vi "Execute.vi"(8 "error in (no error)":errorcluster, 11 "Start Pre-Soak in":refnum<class "Initialize HMI.lvclass">) -> (0 "error out":errorcluster, 3 "Start Pre-Soak out":refnum<class "Initialize HMI.lvclass">)   [LabVIEW 2019, in "Initialize HMI.lvclass"]
uses:
  <vilib>/gpm_packages/@cs/Car-wash/Source/Process Steps/Initialize HMI/Initialize HMI.lvclass
  C:/Program Files/National Instruments/LabVIEW 2019/vi.lib/gpm_packages/@cs/mva-core/Source/IModel/IModel/IModel.lvclass
  C:/Program Files/National Instruments/LabVIEW 2019/vi.lib/ActorFramework/Actor/Actor.lvclass
  <vilib>/gpm_packages/@cs/mva-core/Source/IObserver/IObserver/IObserver.lvclass/IObserver.ctl
  <vilib>/gpm_packages/@cs/mva-core/Source/IModel/IModel/IModel.lvclass/IModel.ctl
  <vilib>/gpm_packages/@cs/mva-core/Source/IMediator/PublishRequest/PublishRequest.lvclass/PublishRequest.ctl
  <vilib>/gpm_packages/@cs/mva-core/Source/IMediator/IMediator Messages/Publish Msg/Publish Msg.lvclass/Publish Msg.ctl
  <vilib>/gpm_packages/@cs/actor-framework-messages/Source/RoundTripMessage/RoundTripMessage.lvclass/RoundTripMessage.ctl
  <vilib>/ActorFramework/Message Enqueuer/Message Enqueuer.lvclass/Message Enqueuer.ctl
  <vilib>/ActorFramework/Actor/Actor.lvclass/Actor.ctl
  <vilib>/gpm_packages/@cs/mva-core/Source/IMediator/IMediator Messages/Publish Msg/Send Pre-Addressed Publish.vi
  <vilib>/gpm_packages/@cs/mva-core/Source/IObserver/IObserver/Read Unique ID.vi
  <vilib>/gpm_packages/@cs/mva-core/Source/IMediator/PublishRequest/Pack Publish Request.vi
  <vilib>/ActorFramework/Message Enqueuer/Init from Existing Queue.vi
  <vilib>/ActorFramework/Message Enqueuer/Enqueue.vi
  <vilib>/gpm_packages/@cs/actor-framework-messages/Source/RoundTripMessage/Return Round-Trip Message.vi
  <vilib>/gpm_packages/@cs/mva-core/Source/IModel/IModel/IModel.lvclass
  C:/Program Files/National Instruments/LabVIEW 2019/vi.lib/gpm_packages/@cs/mva-core/Source/IObserver/IObserver/IObserver.lvclass
  <vilib>/gpm_packages/@cs/mva-core/Source/IMediator/IMediator Messages/Publish Msg/Publish Msg.lvclass
  C:/Program Files/National Instruments/LabVIEW 2019/vi.lib/gpm_packages/@cs/actor-framework-messages/Source/RoundTripMessage/RoundTripMessage.lvclass
  <vilib>/gpm_packages/@cs/actor-framework-messages/Source/RoundTripMessage/RoundTripMessage.lvclass
  C:/Program Files/National Instruments/LabVIEW 2019/vi.lib/ActorFramework/Message/Message.lvclass
  <vilib>/ActorFramework/Stop Msg/Stop Msg.lvclass
  <vilib>/Utility/error.llb/Error Cluster From Error Code.vi
  <vilib>/ActorFramework/Message Priority Queue/Priority Enqueue.vi
  <vilib>/gpm_packages/@cs/mva-core/Source/IMediator/PublishRequest/PublishRequest.lvclass
  <vilib>/ActorFramework/Message Enqueuer/Message Enqueuer.lvclass
  <vilib>/ActorFramework/Actor/Actor.lvclass
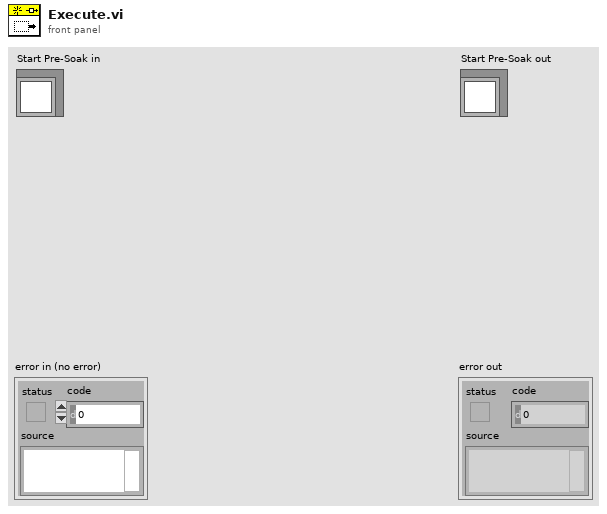
[diagram p1: front panel]
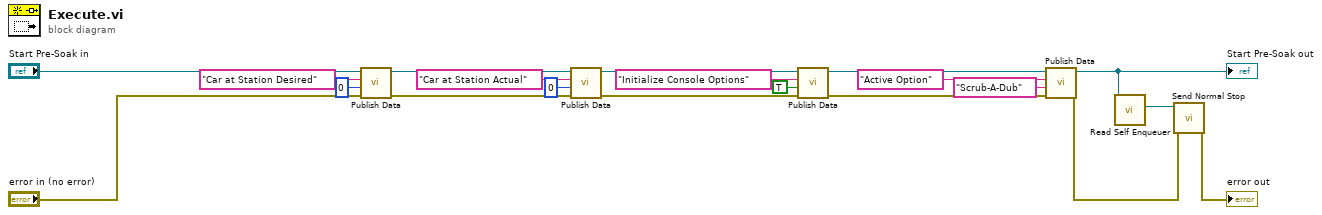
[diagram p0: block diagram]
diagram:
  n1 = call <vilib>:"Publish Data.vi"("error in (no error)"="error in (no error)", "Data to Publish"=u8 0, "Datum Name"="Car at Station Desired", "IModel in"="Start Pre-Soak in") -> ("error out"=w3:errorcluster, "IModel out"=w4:refnum<class "Initialize HMI.lvclass">)  [unwired: 6 in]
  n2 = call <vilib>:"Publish Data.vi"("error in (no error)"=w3, "Data to Publish"=u8 0, "Datum Name"="Car at Station Actual", "IModel in"=w4) -> ("error out"=w9:errorcluster, "IModel out"=w10:refnum<class "Initialize HMI.lvclass">)  [unwired: 6 in]
  n3 = call <vilib>:"Publish Data.vi"("error in (no error)"=w9, "Data to Publish"=TRUE, "Datum Name"="Initialize Console Options", "IModel in"=w10) -> ("error out"=w7:errorcluster, "IModel out"=w8:refnum<class "Initialize HMI.lvclass">)  [unwired: 6 in]
  n4 = call <vilib>:"Publish Data.vi"("error in (no error)"=w7, "Data to Publish"="Scrub-A-Dub", "Datum Name"="Active Option", "IModel in"=w8) -> ("error out"=w13:errorcluster, "IModel out"=w14:refnum<class "Initialize HMI.lvclass">)  [unwired: 6 in]
  "Start Pre-Soak out" <- w14
  n5 = call <vilib>:"Read Self Enqueuer.vi"("Actor"=w14) -> ("Self Enqueuer"=w20:refnum<class "Message Enqueuer.lvclass">)  [unwired: 10 in]
  n6 = call <vilib>:"Send Normal Stop.vi"("error in (no error)"=w13, "Message Enqueuer"=w20) -> ("error out"=→"error out":errorcluster)  [unwired: 9 in]
